vi "Queue Self Alias.vi"(11 "Base Queue jettl in":refnum<class "Base Queue jettl.lvclass">) -> (2 "Queue Self Alias":string)   [LabVIEW 2021, in "jettl.lvlib" / "Base Queue jettl.lvlib" / "Base Queue jettl.lvclass"]
uses:
  Base Queue jettl.lvclass
  Base Queue jettl.lvclass/Base Queue jettl.ctl
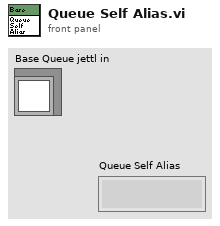
[diagram p1: front panel]
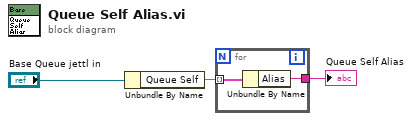
[diagram p0: block diagram]
diagram:
  n1 = Unbundle By Name("Base Queue jettl in") -> ("Queue Self"=w2:map{string, refnum<data-value>})
  n2 = for {
    tunnel: w2 -> [w5] mode=indexing
    tunnel: [w4] -> w1
    n3 = Unbundle By Name(w5) -> ("Alias"=w4:string)
  }
  "Queue Self Alias" <- w1
